vi "Retrieve Async Section configuration properties (objects).vi"(8 "error in":errorcluster, 11 "section item ref in":T2 format="%.0x") -> (0 "error out":errorcluster, 1 "status channel configuration":map{string, map{string, i32}}(c390), 2 "configuration properties":T1[](array[typedef]), 3 "section item ref out":T2 format="%.0x", 4 "Found":bool)   [LabVIEW 2019, in "HLA Custom Device System Explorer.lvlib"]
uses:
  HLA Custom Device System Explorer.lvlib
  <vilib>/NI VeriStand/Custom Device API/Custom Device Item Ref.ctl
  Shared/object_attribute_configuration.ctl
  Shared/Constants.vi
  <vilib>/NI VeriStand/Custom Device API/Get Item Property (String).vi
  <vilib>/NI VeriStand/Custom Device API/Custom Device API.lvlib
  Shared/HLA Custom Device Shared.lvlib
  <vilib>/NI VeriStand/Custom Device Tools/Custom Device Utility Library/Custom Device Utility Library.lvlib
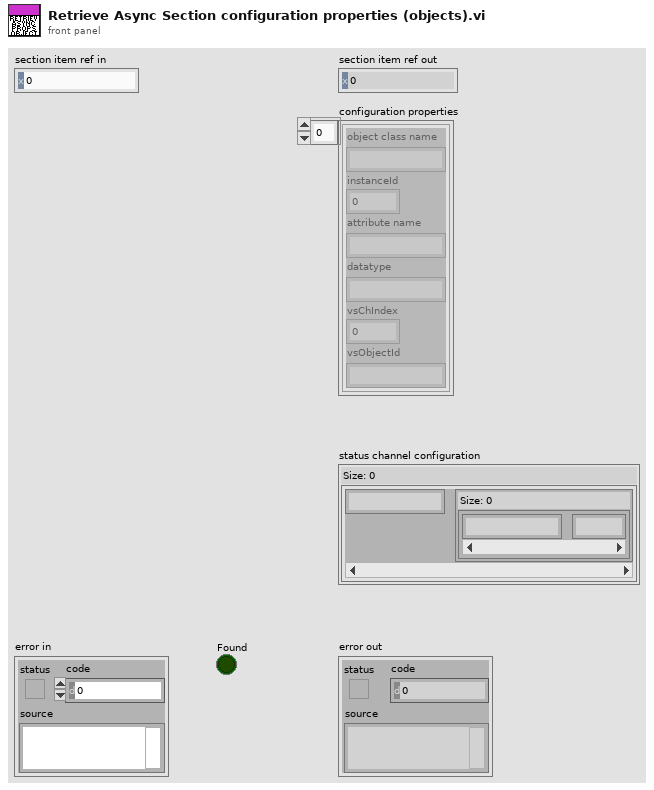
[diagram p1: front panel]
types:
  T1 = typedef "HLA Custom Device Shared.lvlib/object_attribute_configuration.ctl" = cluster{"object class name":string, "instanceId":i32, "attribute name":string, "datatype":string, "vsChIndex":i32, "vsObjectId":string}
  T2 = typedef "Custom Device API.lvlib/Custom Device Item Ref.ctl" = u64
  T3 = typedef "Custom Device API.lvlib/Custom Device Item Info.ctl" = cluster{"Name":string, "Is Channel":bool, "GUID":string, "Is Waveform":bool}
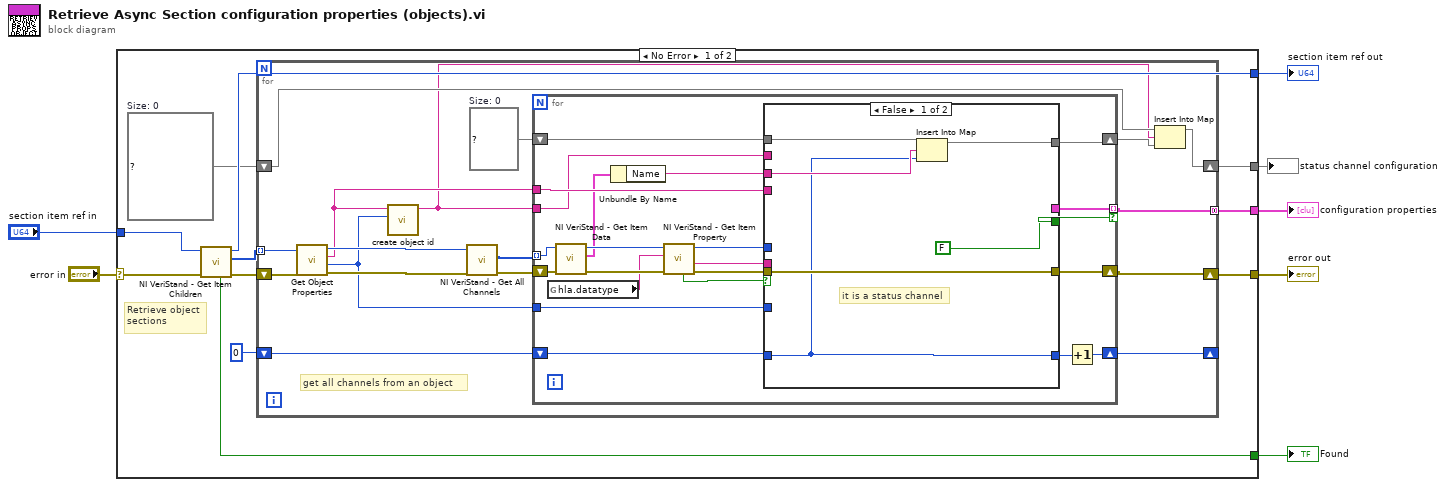
[diagram p0: block diagram]
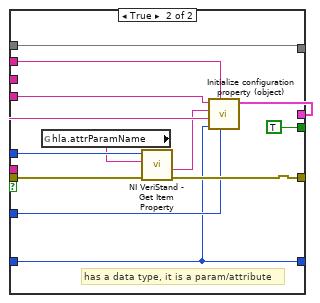
[diagram p2: hidden frame]
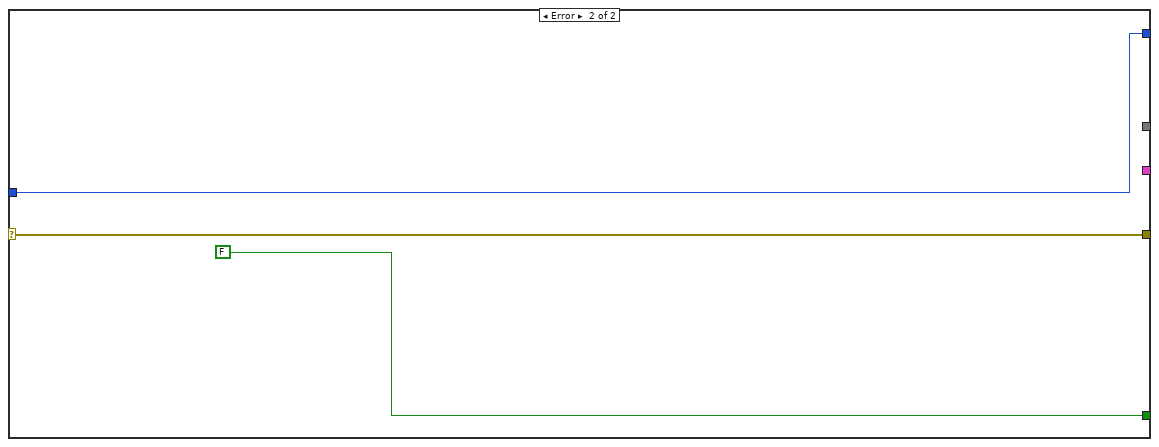
[diagram p3: hidden frame]
diagram:
  n1 = case shown="No Error" "error in" {
    selector: "error in" -> [w15 w78]
    tunnel: [w14 w78] -> w6
    tunnel: [w13 w79] -> w5
    tunnel: "section item ref in" -> [w16 w79]
    tunnel: [w11 FALSE ("Found")] -> w3
    tunnel: [w12 _] -> w2
    tunnel: [w9 _] -> w1
    frame No Error {
      w10 = map{string, map{string, i32}} {}  # Size: 0
      # "Retrieve object\nsections"
      n2 = call <vilib>:"NI VeriStand - Get Item Children.vi"("error in (no error)"=w15, "Item Ref in"=w16) -> ("error out"=w17:errorcluster, "Child Refs"=w18:T2[], "Item Ref out"=w13:T2, "Found"=w11:bool)  [unwired: 6 in]
      n3 = for {
        shift-right: [w28] -> w14
        shift-left: w17 -> [w35]
        tunnel: w18 -> [w34] mode=indexing
        tunnel: [w29] -> w12 mode=concatenating
        shift-right: [w30] -> w9
        shift-left: w10 -> [w32]
        shift-right: [w19] -> _
        shift-left: 0 -> [w20]
        w33 = map{string, i32} {}  # Size: 0
        # "get all channels from an object"
        n4 = call "Get Object Properties.vi"("error in (no error)"=w35, "Item Ref in"=w34) -> ("error out"=w24:errorcluster, "instance id"=w22:i32, "class name"=w23:string, "Item Ref out"=w25:T2)  [unwired: 6 in]
        n5 = call "create object id.vi"("instance id (0)"=w22, "class name"=w23) -> ("String"=w21:string)  [unwired: 9 in]
        n6 = call <vilib>:"NI VeriStand - Get All Channels.vi"("error in"=w24, "Section Ref in"=w25) -> ("error out"=w26:errorcluster, "Channel Refs"=w27:T2[])  [unwired: 6 in, 2 out]
        n7 = for {
          tunnel: w23 -> [w52]
          tunnel: w27 -> [w57] mode=indexing
          tunnel: [w51] -> w29 mode=indexing if=w44
          shift-right: [w40] -> w28
          shift-left: w26 -> [w56]
          shift-right: [w45] -> w31
          shift-left: w33 -> [w46]
          tunnel: w22 -> [w43]
          tunnel: w21 -> [w39]
          shift-right: [w38] -> w19
          shift-left: w20 -> [w37]
          n8 = global read "Constants.vi" "hla.datatype"() -> (w53:string)
          n9 = call <vilib>:"NI VeriStand - Get Item Data.vi"("error in (no error)"=w56, "Item Ref in"=w57) -> ("error out"=w54:errorcluster, "Item Info"=w49:T3, "Item Ref out"=w55:T2)  [unwired: 6 in, 1 out]
          n10 = Unbundle By Name(w49) -> ("Name"=w48:string)
          n11 = call-poly <vilib>:"NI VeriStand - Get Item Property.vi"("error in (no error)"=w54, "Property Name"=w53, "Item Ref in"=w55) -> ("error out"=w41:errorcluster, "Value"=w50:string, "Item Ref out"=w42:T2, "Found?"=w47:bool)  [unwired: 5 in]
          n12 = case shown="False" w47 {
            tunnel: w52 -> [_ w66]
            tunnel: [_ w76] -> w51
            tunnel: w50 -> [_ w68]
            tunnel: w48 -> [w62 _]
            tunnel: w46 -> [w63 w74]
            tunnel: w37 -> [w58 w64]
            tunnel: [w61 w74] -> w45
            tunnel: [FALSE TRUE] -> w44
            tunnel: w43 -> [_ w69]
            tunnel: w42 -> [_ w73]
            tunnel: w41 -> [w59 w72]
            tunnel: [w59 w70] -> w40
            tunnel: w39 -> [_ w65]
            tunnel: [w58 w64] -> w36
            frame False {
              # "it is a status channel"
              n13 = Insert Into Map(map in=w63, key=w62, value=w58) -> (map out=w61:map{string, i32})  [unwired: 2 out]
            }
            frame True {
              # "has a data type, it is a param/attribute"
              n14 = global read "Constants.vi" "hla.attrParamName"() -> (w71:string)
              n15 = call-poly <vilib>:"NI VeriStand - Get Item Property.vi"("error in (no error)"=w72, "Property Name"=w71, "Item Ref in"=w73) -> ("error out"=w70:errorcluster, "Value"=w67:string)  [unwired: 5 in, 2 out]
              n16 = call "Initialize configuration property (object).vi"("instance id"=w69, "vsObjectId"=w65, "vsChIndex"=w64, "datatype"=w68, "attribute name"=w67, "class name"=w66) -> ("attribute configuration"=w76:T1)  [unwired: 5 in]
            }
          }
          n17 = Increment(x=w36) -> (x+1=w38:i32)
        }
        n18 = Insert Into Map(map in=w32, key=w21, value=w31) -> (map out=w30:map{string, map{string, i32}})  [unwired: 2 out]
      }
    }
    frame Error {
    }
  }
  "error out" <- w6
  "section item ref out" <- w5
  "Found" <- w3
  "configuration properties" <- w2
  "status channel configuration" <- w1
